vi "Exp_GetFrames.vi"(8 "error in (no error)":errorcluster, 11 "LightField Automation in":refnum<class "LightField Automation.lvclass">) -> (0 "error out":errorcluster, 2 "Frames":i32, 3 "LightField Automation out":refnum<class "LightField Automation.lvclass">)   [LabVIEW 2013, in "LightField Automation.lvclass"]
uses:
  LightField Automation.lvclass
  C:/Program Files/Princeton Instruments/LightField/PrincetonInstruments.LightFieldAddInSupportServices.dll
  Program Files/Princeton Instruments/LightField/PrincetonInstruments.LightFieldAddInSupportServices.dll
  LightField Automation.lvclass/LightField Automation.ctl
  C:/Program Files/Princeton Instruments/LightField/AddInViews/PrincetonInstruments.LightFieldViewV3.dll
  Program Files/Princeton Instruments/LightField/AddInViews/PrincetonInstruments.LightFieldViewV3.dll
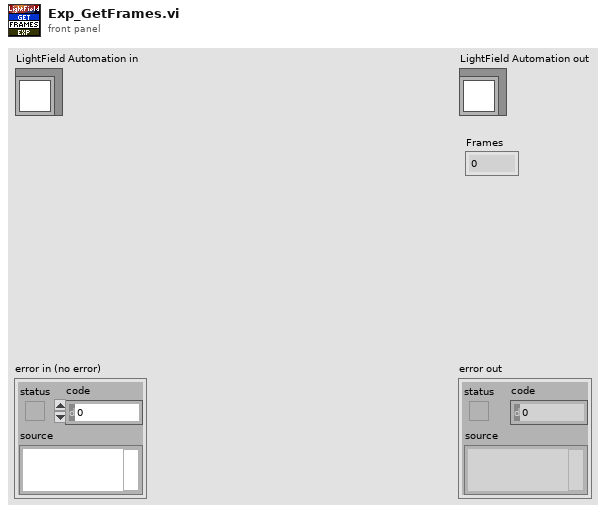
[diagram p1: front panel]
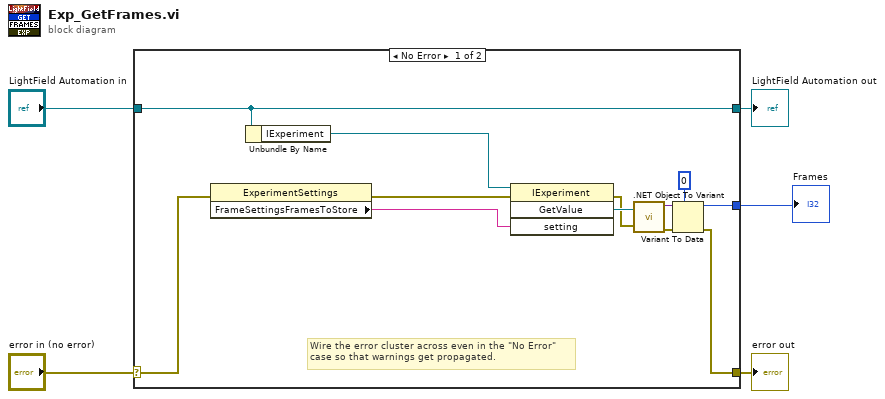
[diagram p0: block diagram]
diagram:
  n1 = case shown="No Error" "error in (no error)" {
    selector: "error in (no error)" -> [w10 w19]
    tunnel: [w6 w19] -> w4
    tunnel: [w9 w18] -> w2
    tunnel: "LightField Automation in" -> [w9 w18]
    tunnel: [w7 _] -> w1
    frame No Error {
      # "Wire the error cluster across even in the \"No Error\"\ncase so that warnings get propagated."
      n2 = property class="ExperimentSettings"(error in=w10) -> (error out=w11:errorcluster, "FrameSettingsFramesToStore"=w12:string)  [unwired: 1 in, 1 out]
      n3 = Unbundle By Name(w9) -> ("IExperiment"=w8:refnum<k24>)
      n4 = invoke class="IExperiment" method="GetValue"(reference=w8, error in=w11, "setting"=w12) -> (error out=w13:errorcluster, "GetValue"=w14:refnum<k24>)  [unwired: 1 in, 2 out]
      n5 = call <vilib>:".NET Object To Variant.vi"("error in (no error)"=w13, ".NET object"=w14) -> ("error out"=w17:errorcluster, "variant"=w15:variant)
      n6 = Variant To Data(error in=w17, type=0, Variant=w15) -> (data=w7:i32, error out=w6:errorcluster)
    }
    frame Error {
    }
  }
  "error out" <- w4
  "LightField Automation out" <- w2
  "Frames" <- w1
